vi "recive_data_frame.vi"(0 "VISA resource name out":refnum<visa-resource-name>, 1 "错误输入（无错误）":errorcluster) -> (2 "VISA resource name out 2":refnum<visa-resource-name>, 3 "字符串":string, 4 "error out":errorcluster)   [LabVIEW 2018]
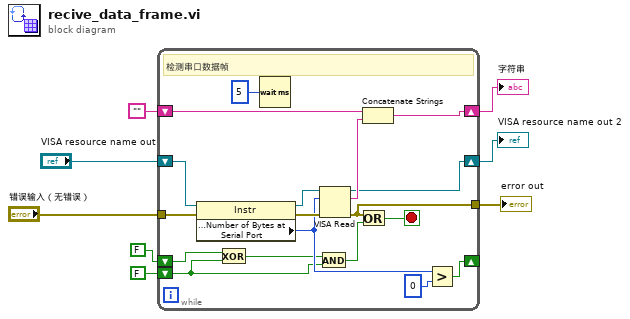
[diagram p0: block diagram]
diagram:
  n1 = while "While循环" {
    tunnel: [w13] -> w2
    shift-right: [w22] -> w1
    shift-left: "" -> [w21]
    shift-right: [w17] -> _
    shift-left: FALSE -> [w16]
    shift-left: FALSE -> [w14]
    shift-right: [w23] -> w3
    shift-left: "VISA resource name out" -> [w10]
    tunnel: "错误输入（无错误）" -> [w9]
    stop <- w11 stop-if-true
    # "检测串口数据帧"
    n2 = property class="Instr"(reference=w10, error in=w9) -> (reference out=w25:refnum<visa-resource-name>, error out=w26:errorcluster, "Serial Settings:Number of Bytes at Serial Port"=w19:u32)
    n3 = Exclusive Or(1:w14, 2:w16) -> (0:w15:bool)
    n4 = Wait (ms)(milliseconds to wait=u32 5 ("等待时间（毫秒）")) -> ()  [unwired: 1 out]
    n5 = And(x=w15, y=w14) -> (x .and. y?=w12:bool)
    n6 = VISA Read(VISA resource name=w25, byte count=w19, error in (no error)=w26) -> (VISA resource name out=w23:refnum<visa-resource-name>, read buffer=w24:string, error out=w13:errorcluster)  [unwired: 1 out]
    n7 = Or(x=w13, y=w12) -> (x .or. y?=w11:bool)
    n8 = Concatenate Strings(w21, w24) -> (w22:string)
    n9 = Greater?(x=w19, y=u32 0) -> (0:w17:bool)
  }
  "VISA resource name out 2" <- w3
  "error out" <- w2
  "字符串" <- w1
